vi "2401 Read Data.vi"() -> (1 "Resistance":dbl, 2 "Current":dbl, 3 "Voltage":dbl)   [LabVIEW 2011]
panel:
  out "Timestamp":dbl
  out "read buffer":string
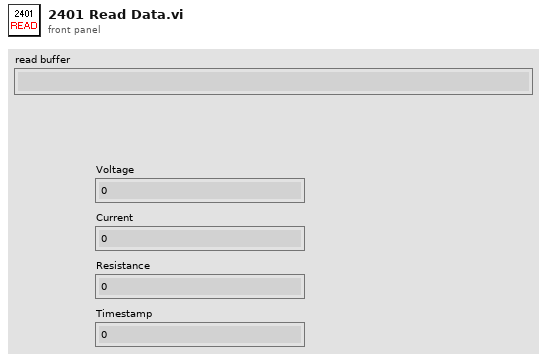
[diagram p1: front panel]
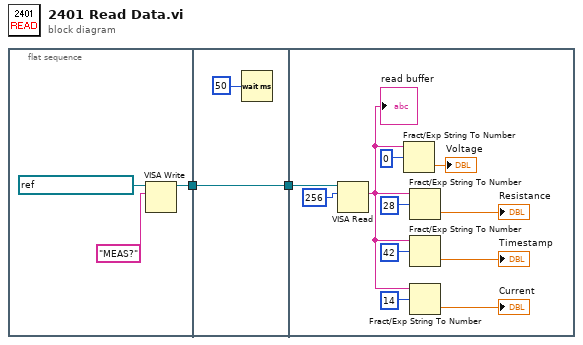
[diagram p0: block diagram]
diagram:
  n1 = flat-sequence {
    tunnel: [w4] -> w2
    tunnel: w2 -> [w7]
    tunnel: [w7] -> w1
    tunnel: w1 -> [w17]
    frame #0 {
      n2 = VISA Write(VISA resource name=refnum<visa-resource-name> "GPIB0::13::INSTR", write buffer="MEAS?") -> (VISA resource name out=w4:refnum<visa-resource-name>)  [unwired: 1 in, 2 out]
    }
    frame #1 {
      n3 = Wait (ms)(milliseconds to wait=u32 50) -> ()  [unwired: 1 out]
    }
    frame #2 {
      n4 = VISA Read(VISA resource name=w17, byte count=u32 256) -> (read buffer=w16:string)  [unwired: 1 in, 3 out]
      "read buffer" <- w16
      n5 = Fract/Exp String To Number(string=w16, offset=0) -> (number=→"Voltage":dbl)  [unwired: 2 in, 1 out]
      n6 = Fract/Exp String To Number(string=w16, offset=28) -> (number=→"Resistance":dbl)  [unwired: 2 in, 1 out]
      n7 = Fract/Exp String To Number(string=w16, offset=42) -> (number=→"Timestamp":dbl)  [unwired: 2 in, 1 out]
      n8 = Fract/Exp String To Number(string=w16, offset=14) -> (number=→"Current":dbl)  [unwired: 2 in, 1 out]
    }
  }
